vi "Write Test Period.vi"(8 "error in (no error)":errorcluster, 10 "test period":dbl, 11 "Ramp Setpoint in":refnum<class "Ramp Setpoint.lvclass">) -> (0 "error out":errorcluster, 3 "Ramp Setpoint out":refnum<class "Ramp Setpoint.lvclass">)   [LabVIEW 2020, in "Ramp Setpoint.lvclass"]
uses:
  Ramp Setpoint.lvclass
  Ramp Setpoint.lvclass/Ramp Setpoint.ctl
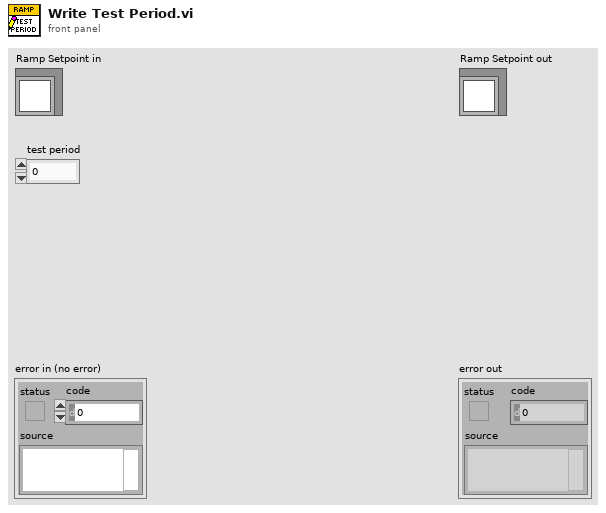
[diagram p1: front panel]
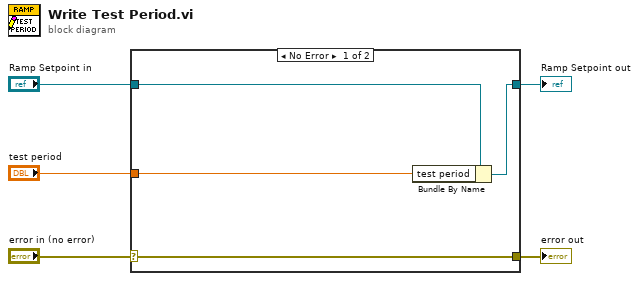
[diagram p0: block diagram]
diagram:
  n1 = case shown="No Error" "error in (no error)" {
    selector: "error in (no error)" -> [w9 w10]
    tunnel: [w9 w10] -> w4
    tunnel: [w7 w11] -> w2
    tunnel: "Ramp Setpoint in" -> [w8 w11]
    tunnel: "test period" -> [w6 _]
    frame No Error {
      n2 = Bundle By Name(cluster=w8, "test period"=w6) -> (w7:refnum<class "Ramp Setpoint.lvclass">)
    }
    frame Error {
    }
  }
  "error out" <- w4
  "Ramp Setpoint out" <- w2
